vi "Find Center.vi"(5 "Position":i32, 7 "Tray Number":dbl format="%#_13g", 8 "Assembly Type":string, 9 "XYZTheta":dbl[](array[numeric]), 10 "component thickness":dbl, 11 "Gantry In":refnum<k24>) -> (0 "Pedestal Heights":dbl[][](array[numeric]), 1 "XYZTheta Centers":dbl[][](array[numeric]), 3 "Gantry Out":refnum<k24>)   [LabVIEW 2021, in "Assembly Tray.lvclass"]
uses:
  Assembly Tray.lvclass
  Find Tray.ctl
  Controller/Camera/Machine Vision.ctl
  C:/Program Files (x86)/Aerotech/A3200/LabVIEW/2010/Bin/Aerotech.A3200.dll
  Program Files (x86)/Aerotech/A3200/LabVIEW/2010/Bin/Aerotech.A3200.dll
  Controller/Camera/Image processing.ctl
  Controller/Camera/Camera settings.ctl
  <vilib>/Utility/file.llb/Read Delimited Spreadsheet (DBL).vi
  Controller/Camera/Camera.lvclass
  Controller/Motion/A3200/A3200.lvclass
  Controller/Motion/Motion.lvclass
  <vilib>/vision/NI_Vision_Development_Module.lvlib
panel:
  out "Global Report.Standard Variation":sgl
  in  "BP check":bool
  out "Program Done?":bool
  out "Manual Mode?":bool
  in  "Enter Manual Mode":bool
  out "error out":errorcluster
  out "Radius (Real-World)":dbl
  out "Match found?":bool
  out "Distance as expected?":bool
  in  "Auto Submit":bool
  out "Instructions":string="Use the joystick to match the pattern recognition until a red circle appears.\nUse Z controls to focus if needed."
  out "resulting string":string
  out "Current Z High Speed":dbl
  out "Current XY High Speed":dbl
  out "current Z low speed":dbl
  out "current XY speed":dbl
  in  "Z high":dbl=12.5
  in  "XY high":dbl=50.0
  in  "Z low":dbl=0.05
  in  "XY low":dbl=0.1
  out "Low Speed":bool
  out "X":bool
  out "Y":bool
  out "Z":bool
  out "High Speed":bool
  out "Move by":dbl[](array[numeric])
  in  "Autofiducial (Beta)":bool
  out "maximum is best focus":dbl
  in  "Focus":bool
  in  "Camera settings":T1={"Gamma"=1.6, "Gain"=0, "Sharpness"=0, "Contrast"=0.0, "Exposure"=0.0078125} {"Exposure" min=0.000244140625 max=0.5 scale=0.0002..0.5; "Contrast" min=0.0 max=1.0 scale=0.001..1.0; "Sharpness" min=0 max=2 step=1 scale=0.0..2.0; "Gain" min=0 max=100 step=1 scale=0.1..100.0; "Gamma" min=0.01 max=10.0 scale=0.01..10.0}
  in  "Image processing":T2={"Brightness"=128.0, "Contrast"=45.0, "Gamma"=1.0471123} {"Brightness" scale=0.0..400.0; "Contrast" scale=0.0..90.0; "Gamma" scale=0.005..5.0}
  in  "Override camera presets":bool
  out "Both fiducials recorded":bool
  in  "Machine Vision":T3
  out "Right Fiducial":dbl[](array[numeric]) format="%.6g"
  out "Left Fiducial":dbl[](array[numeric]) format="%.6g"
  out "Gantry":dbl[](array[numeric]) format="%.6g"
  out "Sum":dbl[](array[numeric]) format="%.6g"
  out "Camera":dbl[](array[numeric]) format="%.6g"
  in  "Carrier Tray":T4
  out "Image":T5(plugin-control)
  out "Center":dbl[](array[numeric]) format="%.6g"
  in  "Position Number":i16=1
  in  "Go to Center":bool
  in  "Calculate":bool
  in  "Record Top Right":bool
  in  "Record Top Left":bool
  in  "Go to Top Right Fiducial":bool
  in  "Go to Top Left Fiducial":bool
  in  "Joystick":bool
  in  "Stop":bool
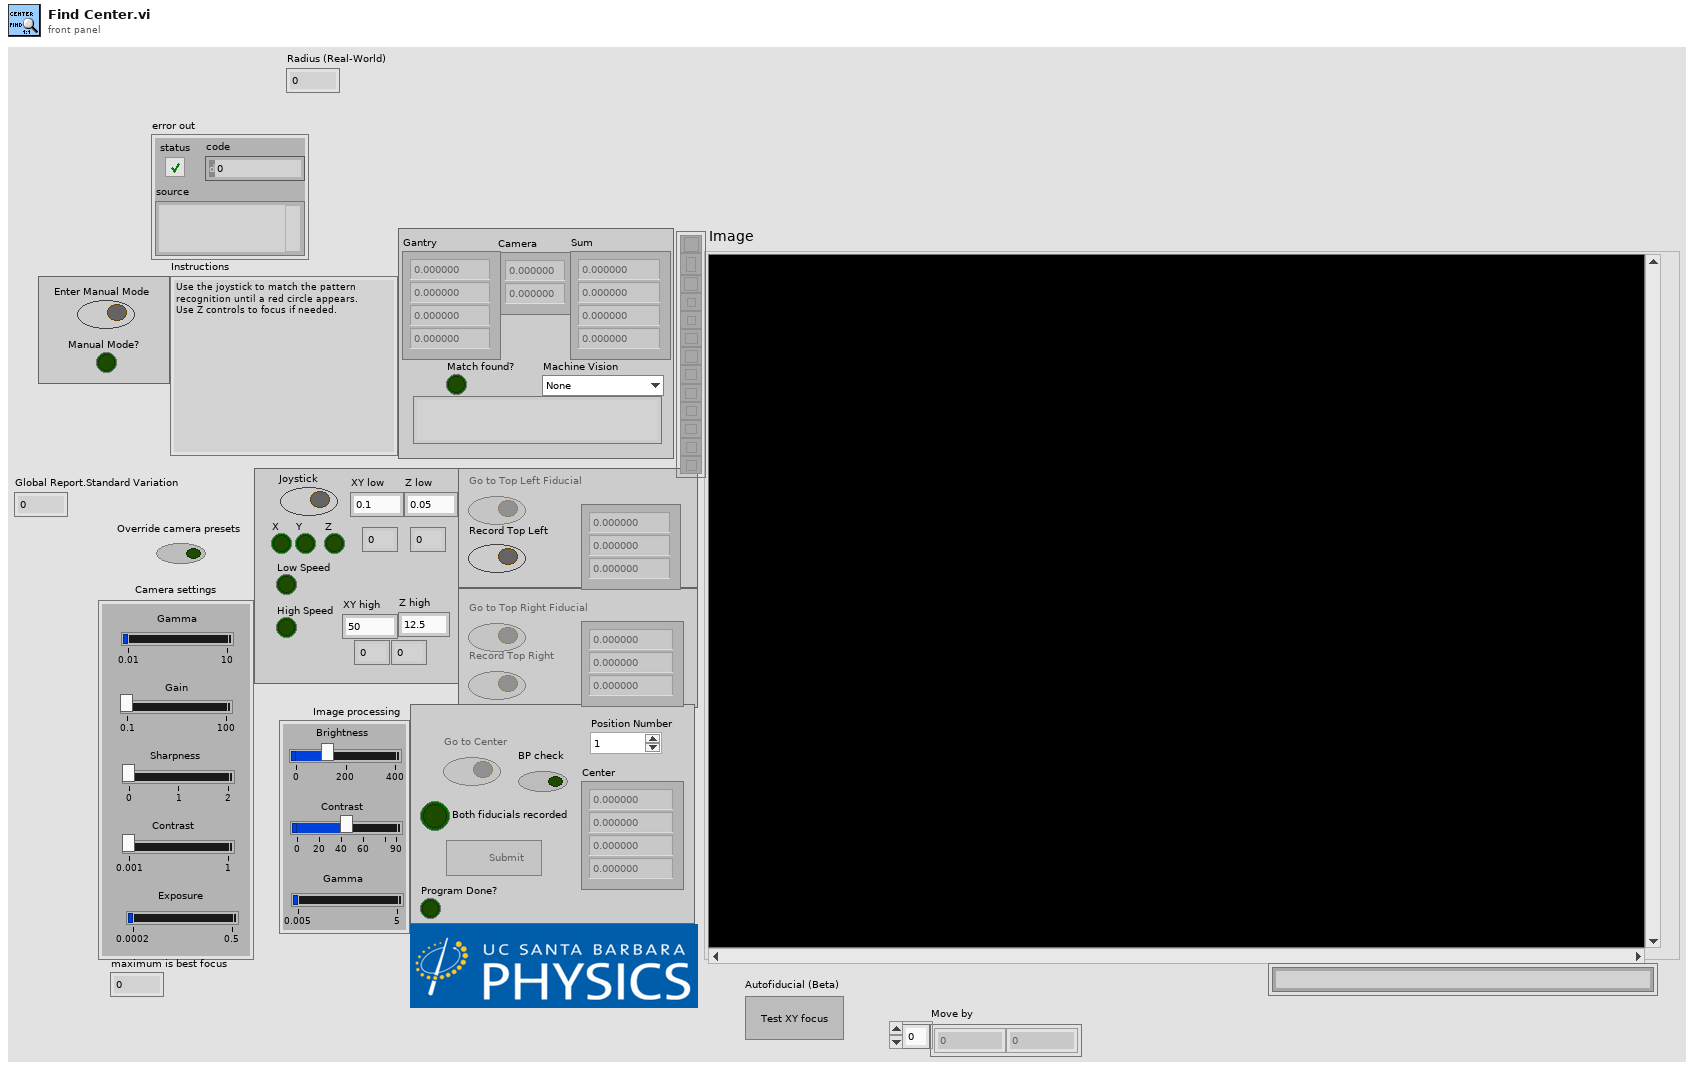
[diagram p1: front panel]
types:
  T1 = typedef "Camera.lvclass/Camera settings.ctl" = cluster{"Gamma":dbl, "Gain":i64, "Sharpness":i64, "Contrast":dbl, "Exposure":dbl}
  T2 = typedef "Camera.lvclass/Image processing.ctl" = cluster{"Brightness":sgl, "Contrast":sgl, "Gamma":sgl}
  T3 = typedef "Camera.lvclass/Machine Vision.ctl" = enum16{"None", "Assembly Tray Circle", "Assembly Tray Fiducial", "Partial Hexaboard", "sensor edge init", "HB edge init", "sensor edge pos1", "sensor edge pos2", "HB edge pos1", "HB edge pos2", "Sensor CH1-2", "HB CH1", "HB CH2", "V3 Sensor Circle", "Hexaboard Circle", "sensor CH1 check", "HB CH1 check ", "sensor ID"}
  T4 = typedef "Assembly Tray.lvclass/Find Tray.ctl" = cluster{"Gantry Fiducials":dbl[], "Relative Coordinates":dbl[][], "Camera Fiducials":dbl[][], "XYZTheta Centers":dbl[][], "Workspace Center":dbl[], "Syringe Relative Coordinates":dbl[], "Gantry Region":dbl, "Fiducials":path, "New Fiducials":dbl[][], "Past Fiducials":dbl[][], "XYZTheta":dbl[], "Pedestal Heights":dbl[][], "Assembly Type":string, "Tray Number":string, "Position":i32, "Protomodule?":bool, "avg value count":dbl[], "Previous Avgs":dbl[][], "Offset pins":dbl[][]}
  T5 = typedef "IMAQ Image.ctl" = refnum<image>
  T6 = cluster{"Average Strength":dbl, "Radius (Real-World)":dbl, "Match found?":bool, "initial angle":sgl, "Global Report":cluster{"Mean Value":sgl, "Standard Variation":sgl, "Minimal Value":sgl, "Maximal Value":sgl, "Area (calibrated)":sgl, "Area (pixels)":u32, "%":sgl, "Calibration Valid":bool}}
  T7 = enum8{"Enabled", "Disabled", "Disabled and Grayed Out"}
  T8 = typedef "File Paths.ctl" = cluster{"Glue Pattern Folder":path, "Carrier Tray Folder":path, "Pick Up Tool Fixture Folder":path, "Components Folder":path, "Bellows Tool Offset.txt":path, "Pick Up Tool Offset.txt":path, "Dispense Tip Offset.txt":path, "Log Files":path, "Gantry Assembly Map.txt":path, "Syringe and offset map.txt":path, "Controllers Folder":path, "Local dbase config":path}
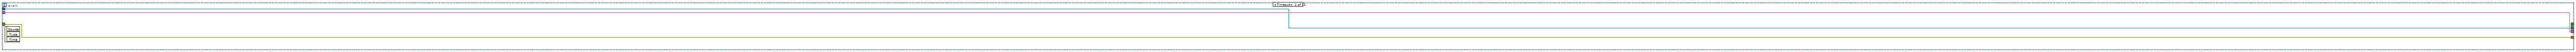
[diagram p3: hidden frame]
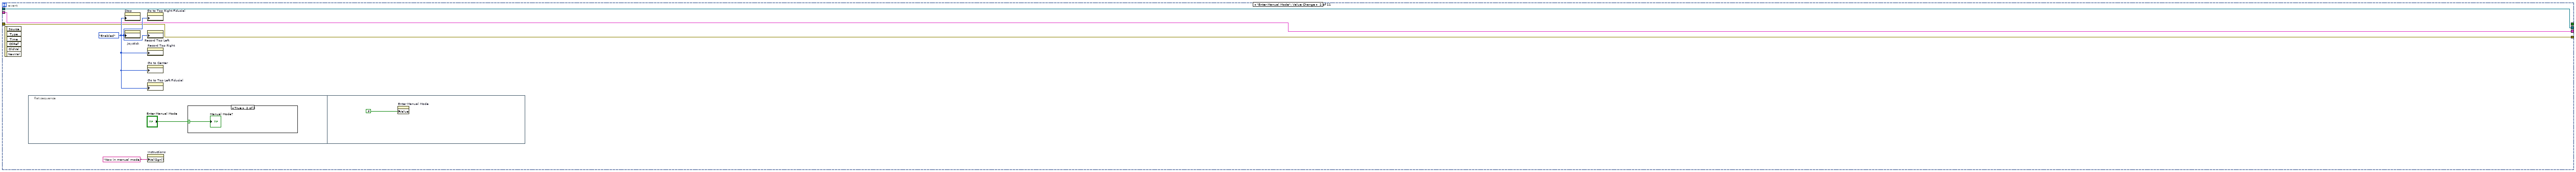
[diagram p4: hidden frame]
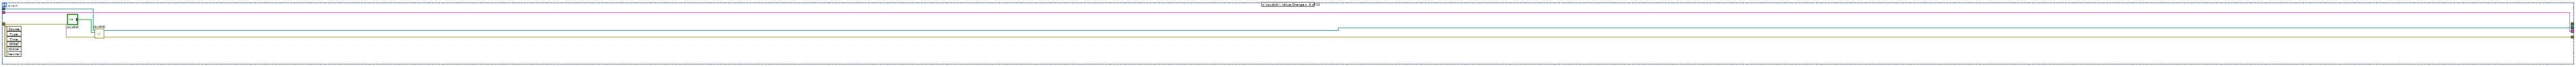
[diagram p6: hidden frame]
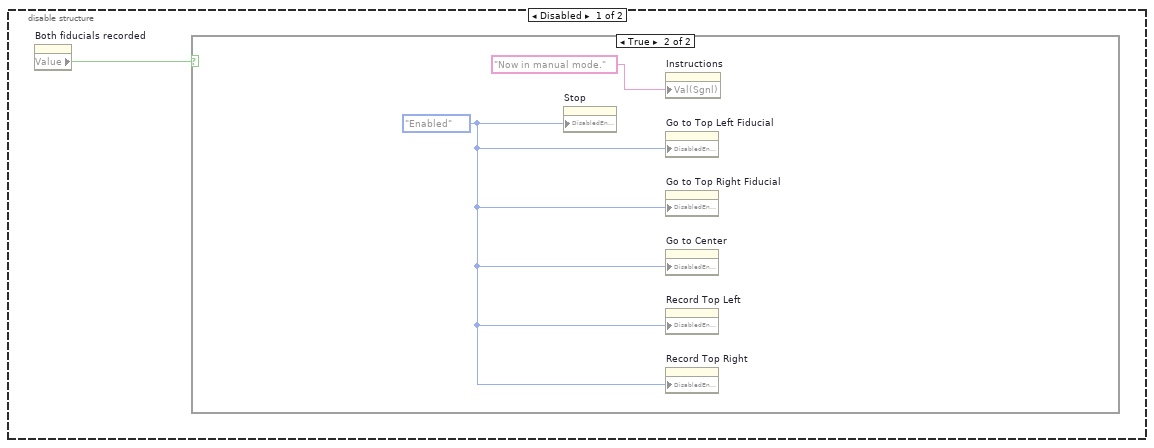
[diagram p7: hidden frame]
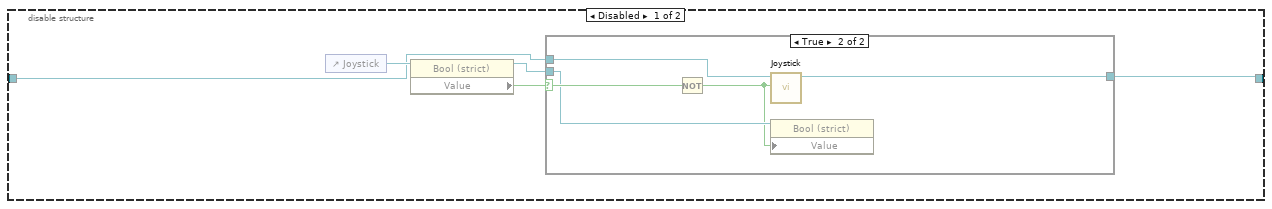
[diagram p9: hidden frame]
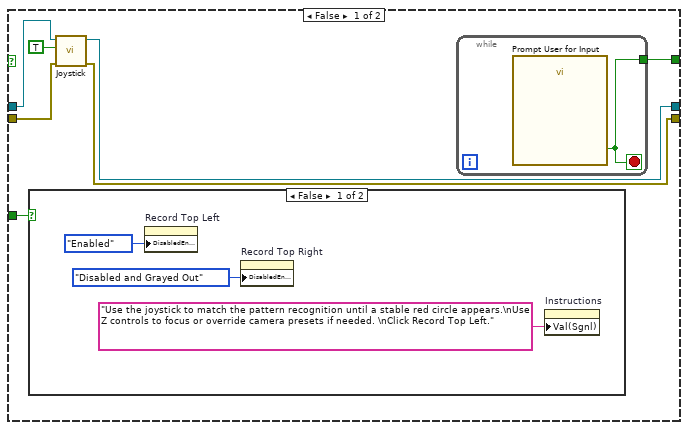
[diagram p12: hidden frame]
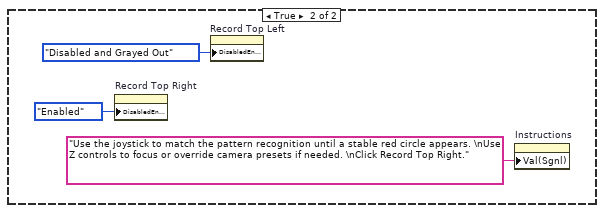
[diagram p13: hidden frame]
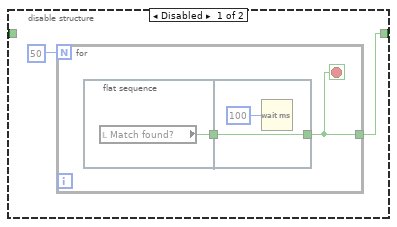
[diagram p19: hidden frame]
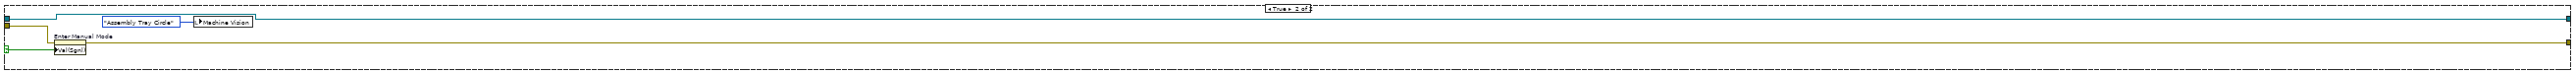
[diagram p20: hidden frame]
diagram:
  n1 = flat-sequence {
    tunnel: [w17] -> w9
    tunnel: ["Gantry In"] -> w8
    tunnel: [w16] -> w7
    tunnel: [w14] -> w4
    tunnel: [w29] -> w5
    tunnel: w9 -> [w29]
    tunnel: [w27] -> w2
    tunnel: w8 -> [w27]
    tunnel: w7 -> [w26]
    tunnel: [w26] -> w6
    tunnel: [w25] -> w1
    tunnel: w4 -> [w24]
    frame #0 {
      n2 = Decrement(x="Position") -> (x-1=w21:i32)
      n3 = call "Find Center Setup.vi"("XYZTheta"="XYZTheta", "Assembly Type"="Assembly Type", "Position"=w21, "Tray Number"="Tray Number", "Carrier Tray"="Carrier Tray") -> ("Assembly Tray Out"=w17:T4)  [unwired: 6 in]
      n4 = call "Get Camera Object.vi"() -> ("error out"=w14:errorcluster, "Camera out"=w16:refnum<class "Camera.lvclass">)  [unwired: 10 in]
    }
    frame #1 {
      n5 = control-ref of="This VI"() -> (w28:refnum<vi>)
      n6 = invoke class="VI" method="Default Vals.Reinit All"(reference=w28, error in=w24) -> (error out=w25:errorcluster)  [unwired: 1 in, 2 out]
    }
  }
  n7 = while {
    shift-right: [w36] -> _
    shift-left: w6 -> [w37]
    tunnel: w2 -> [w34]
    shift-right: [w33] -> _
    shift-left: _ -> [_]
    shift-right: [w31] -> _
    shift-left: w1 -> [w32]
    i -> [w35]
    stop <- w30 stop-if-true
    n8 = flat-sequence {
      tunnel: [w58] -> w36
      tunnel: w34 -> [w44]
      tunnel: [w43] -> w33
      tunnel: w32 -> [w42]
      tunnel: [w41] -> w31
      tunnel: w37 -> [w61]
      tunnel: w35 -> [w56]
      tunnel: [w39] -> w30
      frame #0 {
        n9 = in-place {
          in-place-border: w44 -> [w88]
          in-place-border: [w69] -> w47
          in-place-border: w42 -> [w64]
          in-place-border: [w62] -> w48
          # "Joystck Status"
          n10 = call "Get Joytick Status.vi"("error in (no error)"=w64, "Gantry In"=w88) -> ("error out"=w63:errorcluster, "JoystickLowSpeedActive"=w82:bool, "Joystick Status"=w84:bool[], "Gantry Out"=w70:refnum<k24>, "High Speeds"=w66:dbl[], "Low Speeds"=w65:dbl[])  [unwired: 4 in]
          n11 = Build Array("XY low", "XY low", "XY low", "Z low") -> (w68:dbl[])
          n12 = Build Array("XY high", "XY high", "XY high", "Z high") -> (w67:dbl[])
          n13 = call "Set Joystick Speed.vi"("error in (no error)"=w63, "High Speed Inputs"=w67, "Low Speed Inputs"=w68, "Gantry"=w70) -> ("error out"=w62:errorcluster, "Controller Out"=w69:refnum<k24>)  [unwired: 6 in]
          n14 = Or Array Elements(Boolean array=w84) -> (logical OR=w80:bool)
          n15 = Not(x=w82) -> (.not. x?=w81:bool)
          n16 = Index Array(array=w66) -> (element #1=→"Current XY High Speed":dbl, element #3=→"Current Z High Speed":dbl)  [unwired: 3 in, 1 out]
          n17 = Index Array(array=w65) -> (element #1=→"current XY speed":dbl, element #3=→"current Z low speed":dbl)  [unwired: 3 in, 1 out]
          n18 = Index Array(array=w84) -> (element #1=→"X":bool, element #2=→"Y":bool, element #3=→"Z":bool)  [unwired: 3 in]
          n19 = And(x=w80, y=w82) -> (x .and. y?=→"Low Speed":bool)
          n20 = And(x=w81, y=w80) -> (x .and. y?=→"High Speed":bool)
        }
        n21 = Equal To 0?(x=w56) -> (x = 0?=w55:bool)
        n22 = local read "Program Done?"() -> (w39:bool)
        n23 = call "Camera.vi"("Camera in"=w61, "Stop"=w39, "BCG Image Processing"="Image processing", "Machine Vision"="Machine Vision", "Camera settings"="Camera settings", "Loop 0"=w55, "Override presets"="Override camera presets") -> ("Camera out"=w58:refnum<class "Camera.lvclass">, "output cluster"=w54:T6, "Image"=→"Image":T5, "Camera"=w40:dbl[])  [unwired: 5 in, 4 out]
        "Camera" <- w40
        n24 = call "Get Current Position.vi"("error in (no error)"=w48, "Gantry In"=w47) -> ("error out"=w41:errorcluster, "XYZTheta Out"=w46:dbl[], "Gantry Out"=w43:refnum<k24>)  [unwired: 7 in]
        "Gantry" <- w46
        n25 = Unbundle By Name(w54) -> ("Average Strength"=→"maximum is best focus":dbl, "Radius (Real-World)"=→"Radius (Real-World)":dbl, "Match found?"=→"Match found?":bool, "Global Report.Standard Variation"=w38:sgl)
        "Global Report.Standard Variation" <- w38
        n26 = shared-variable ".\\Assembly Tray.lvclass\\BP Standard Variation"(w38) -> ()  [unwired: 1 in, 1 out]
        n27 = Add(x=w46, y=w40) -> (x+y=→"Sum":dbl[])
      }
    }
  }
  n28 = while {
    shift-right: [w98] -> w13
    shift-left: w5 -> [w99]
    shift-right: [w95] -> w11
    shift-left: w2 -> [w96]
    tunnel: w5 -> [w91]
    shift-right: [w89] -> w3
    shift-left: w1 -> [w90]
    i -> [w94]
    stop <- w97 stop-if-true
    n29 = event shown="[3] \"Go to Top Left Fiducial\", \"Go to Top Right Fiducial\": Value Change" {
      selector: _ -> [_ _ _ _ _ _ _ _ _ _ _]
      dyn-events: _ -> [_ _ _ _ _ _ _ _ _ _ _]
      timeout: _ -> [_ _ _ _ _ _ _ _ _ _ _]
      tunnel: [w111 w114 w125 w143 w366 w425 w563 w711 w789 w809 w882] -> w98
      tunnel: w99 -> [w111 w114 w125 w143 w362 w425 w564 w711 w790 w809 w882]
      tunnel: [_ _ _ _ _ _ _ _ _ w810 _] -> w97
      tunnel: w96 -> [w110 w115 w124 w142 w361 w424 w569 w721 w787 w813 w884]
      tunnel: [w110 w115 w122 w141 w360 w423 w569 w714 w784 w812 w885] -> w95
      tunnel: [w109 w113 w120 w132 w355 w419 w557 w715 w781 w817 w880] -> w89
      tunnel: w90 -> [w109 w113 w121 w133 w357 w418 w560 w720 w781 w814 w881]
      event Timeout {
        n30 = event-data() -> ()  [unwired: 1 in, 3 out]
      }
      event "Enter Manual Mode": Value Change {
        w116 = T7."Enabled" ("Disabled")
        n31 = event-data() -> ()  [unwired: 1 in, 6 out]
        n32 = flat-sequence {
          frame #0 {
            n33 = case shown="True" "Enter Manual Mode" {
              selector: "Enter Manual Mode" -> [_ w118]
              frame False {
              }
              frame True {
                "Manual Mode?" <- w118
              }
            }
          }
          frame #1 {
            n34 = property on="Enter Manual Mode" class="Bool (strict)"("Value"=FALSE ("Enter Manual Mode")) -> ()  [unwired: 2 in, 2 out]
          }
        }
        n35 = property on="Stop" class="Bool"("DisabledEnum"=w116) -> ()  [unwired: 2 in, 2 out]
        n36 = property on="Joystick" class="Bool (strict)"("DisabledEnum"=w116) -> ()  [unwired: 2 in, 2 out]
        n37 = property on="Go to Top Right Fiducial" class="Bool (strict)"("DisabledEnum"=w116) -> ()  [unwired: 2 in, 2 out]
        n38 = property on="Record Top Left" class="Bool (strict)"("DisabledEnum"=w116) -> ()  [unwired: 2 in, 2 out]
        n39 = property on="Record Top Right" class="Bool (strict)"("DisabledEnum"=w116) -> ()  [unwired: 2 in, 2 out]
        n40 = property on="Go to Center" class="Bool"("DisabledEnum"=w116) -> ()  [unwired: 2 in, 2 out]
        n41 = property on="Go to Top Left Fiducial" class="Bool (strict)"("DisabledEnum"=w116) -> ()  [unwired: 2 in, 2 out]
        n42 = property on="Instructions" class="Str"("Val(Sgnl)"="Now in manual mode." ("Value (Signaling)")) -> ()  [unwired: 2 in, 2 out]
      }
      event "Joystick": Value Change {
        n43 = event-data() -> ()  [unwired: 1 in, 6 out]
        n44 = call "Joystick.vi"("error in (no error)"=w121, "Joystick"="Joystick", "Gantry In"=w124) -> ("error out"=w120:errorcluster, "Gantry Out"=w122:refnum<k24>)  [unwired: 7 in]
      }
      event "Go to Top Left Fiducial", "Go to Top Right Fiducial": Value Change {
        n45 = event-data() -> ()  [unwired: 1 in, 6 out]
        n46 = disable-structure shown="Enabled" {
          frame Disabled {
            n47 = property on="Both fiducials recorded" class="Bool (strict)"() -> ("Value"=w144:bool)  [unwired: 2 in, 2 out]
            n48 = case shown="True" w144 {
              frame False {
              }
              frame True {
                w145 = T7."Enabled" ("Disabled")
                n49 = property on="Stop" class="Bool"("DisabledEnum"=w145) -> ()  [unwired: 2 in, 2 out]
                n50 = property on="Instructions" class="Str"("Val(Sgnl)"="Now in manual mode." ("Value (Signaling)")) -> ()  [unwired: 2 in, 2 out]
                n51 = property on="Go to Top Left Fiducial" class="Bool (strict)"("DisabledEnum"=w145) -> ()  [unwired: 2 in, 2 out]
                n52 = property on="Go to Top Right Fiducial" class="Bool (strict)"("DisabledEnum"=w145) -> ()  [unwired: 2 in, 2 out]
                n53 = property on="Go to Center" class="Bool"("DisabledEnum"=w145) -> ()  [unwired: 2 in, 2 out]
                n54 = property on="Record Top Left" class="Bool (strict)"("DisabledEnum"=w145) -> ()  [unwired: 2 in, 2 out]
                n55 = property on="Record Top Right" class="Bool (strict)"("DisabledEnum"=w145) -> ()  [unwired: 2 in, 2 out]
              }
            }
          }
          frame Enabled {
          }
        }
        n56 = disable-structure shown="Enabled" {
          disable-tunnel: w142 -> [w149 w158]
          disable-tunnel: [w147 w158] -> w140
          frame Disabled {
            n57 = control-ref of="Joystick"() -> (w151:refnum<vi>)
            n58 = property class="Bool (strict)"(reference=w151) -> (reference out=w148:refnum<vi>, "Value"=w150:bool)  [unwired: 1 in, 1 out]
            n59 = case shown="True" w150 {
              selector: w150 -> [_ w157]
              tunnel: w149 -> [w152 w155]
              tunnel: [w152 w154] -> w147
              tunnel: w148 -> [_ w156]
              frame False {
              }
              frame True {
                n60 = Not(x=w157) -> (.not. x?=w153:bool)
                n61 = call "Joystick.vi"("Joystick"=w153, "Gantry In"=w155) -> ("Gantry Out"=w154:refnum<k24>)  [unwired: 8 in, 1 out]
                n62 = property class="Bool (strict)"(reference=w156, "Value"=w153) -> ()  [unwired: 1 in, 2 out]
              }
            }
          }
          frame Enabled {
          }
        }
        n63 = Unbundle By Name "Unbundle By Name"(w143) -> ("Gantry Fiducials"=w135:dbl[])
        n64 = flat-sequence {
          tunnel: w135 -> [w160]
          tunnel: w140 -> [w161]
          tunnel: [w161] -> w131
          tunnel: [w160] -> w129
          tunnel: ["Go to Top Right Fiducial"] -> w127
          tunnel: ["Go to Top Right Fiducial"] -> w134
          tunnel: w131 -> [w165]
          tunnel: [w165] -> w130
          tunnel: w129 -> [w164]
          tunnel: [w164] -> w128
          tunnel: w127 -> [w163]
          tunnel: [w163] -> w126
          tunnel: [w183] -> w139
          tunnel: [w179] -> w136
          tunnel: w130 -> [w177]
          tunnel: w128 -> [w174]
          tunnel: w126 -> [w171]
          tunnel: w133 -> [w167]
          tunnel: w139 -> [w185]
          tunnel: [w185] -> w138
          tunnel: [w184] -> w137
          tunnel: w136 -> [w184]
          tunnel: [w188] -> w141
          tunnel: [w187] -> w132
          tunnel: w137 -> [w190]
          tunnel: w134 -> [w191]
          tunnel: w138 -> [w192]
          frame #0 {
          }
          frame #1 {
            w162 = FALSE ("Go to Top Right Fiducial")
            n65 = property on="Go to Top Left Fiducial" class="Bool (strict)"("Value"=w162) -> ()  [unwired: 2 in, 2 out]
            n66 = property on="Go to Top Right Fiducial" class="Bool (strict)"("Value"=w162) -> ()  [unwired: 2 in, 2 out]
          }
          frame #2 {
            w180 = T7."Disabled and Grayed Out" ("Disabled")
            n67 = Select(t=3, s=w171, f=0) -> (s? t:f=w169:i32)
            n68 = call "Joystick.vi"("error in (no error)"=w167, "Joystick"=FALSE, "Gantry In"=w177) -> ("error out"=w175:errorcluster, "Gantry Out"=w178:refnum<k24>)  [unwired: 7 in]
            n69 = Array Subset "Array Subset"(array=w174, index=w169, length=3) -> (w173:dbl[])
            n70 = property on="Instructions" class="Str"("Val(Sgnl)"="Wait for movement to stop." ("Value (Signaling)")) -> ()  [unwired: 2 in, 2 out]
            n71 = property on="Go to Center" class="Bool"("DisabledEnum"=w180) -> ()  [unwired: 2 in, 2 out]
            n72 = property on="Stop" class="Bool"("DisabledEnum"=w180) -> ()  [unwired: 2 in, 2 out]
            n73 = property on="Record Top Right" class="Bool (strict)"("DisabledEnum"=w180) -> ()  [unwired: 2 in, 2 out]
            n74 = property on="Go to Top Right Fiducial" class="Bool (strict)"("DisabledEnum"=w180) -> ()  [unwired: 2 in, 2 out]
            n75 = property on="Go to Top Left Fiducial" class="Bool (strict)"("DisabledEnum"=w180) -> ()  [unwired: 2 in, 2 out]
            n76 = property on="Record Top Left" class="Bool (strict)"("DisabledEnum"=w180) -> ()  [unwired: 2 in, 2 out]
            n77 = local write "Machine Vision"(Machine_Vision."Assembly Tray Fiducial" ("Machine Vision")) -> ()
            n78 = call "ClearXYZTheta Go.vi"("error in (no error)"=w175, "Speed"=300.0, "XYZTheta In"=w173, "Gantry In"=w178) -> ("error out"=w179:errorcluster, "Gantry Out"=w183:refnum<k24>)  [unwired: 5 in, 1 out]
          }
          frame #3 {
            n79 = disable-structure shown="Enabled" {
              frame Enabled {
                n80 = Wait (ms)(milliseconds to wait=u32 500) -> ()  [unwired: 1 out]
              }
              frame Disabled {
              }
            }
          }
          frame #4 {
            n81 = local read "Manual Mode?"() -> (w189:bool)
            n82 = case shown="False" w189 {
              selector: w189 -> [_ w352]
              tunnel: w192 -> [w214 w353]
              tunnel: [w194 w353] -> w188
              tunnel: w191 -> [w195 _]
              tunnel: w190 -> [w213 w351]
              tunnel: [w193 w350] -> w187
              frame False {
                n83 = flat-sequence {
                  tunnel: w214 -> [w239]
                  tunnel: w213 -> [w237]
                  tunnel: [w238] -> w212
                  tunnel: [w236] -> w211
                  tunnel: [w235] -> w210
                  tunnel: [w234] -> w209
                  tunnel: w212 -> [w299]
                  tunnel: w211 -> [w298]
                  tunnel: w210 -> [w297]
                  tunnel: w209 -> [w296]
                  tunnel: [w299] -> w208
                  tunnel: [w298] -> w206
                  tunnel: [w297] -> w204
                  tunnel: [w296] -> w202
                  tunnel: w208 -> [w303]
                  tunnel: [w303] -> w207
                  tunnel: w206 -> [w302]
                  tunnel: [w302] -> w205
                  tunnel: w204 -> [w301]
                  tunnel: [w301] -> w203
                  tunnel: w202 -> [w300]
                  tunnel: [w300] -> w201
                  tunnel: w207 -> [w311]
                  tunnel: w205 -> [w310]
                  tunnel: w203 -> [w306]
                  tunnel: w201 -> [w309]
                  tunnel: [w308] -> w199
                  tunnel: [w307] -> w200
                  tunnel: [w305] -> w196
                  frame #0 {
                    n84 = for {
                      N: 50 -> [_]
                      tunnel: [w242] -> w240
                      tunnel: [w241] -> w232
                      stop <- w242 stop-if-true
                      n85 = flat-sequence {
                        tunnel: [w245] -> w243
                        tunnel: [w244] -> w241
                        tunnel: [w247] -> w242
                        tunnel: w243 -> [w247]
                        frame #0 {
                          n86 = local read "Match found?"() -> (w245:bool)
                          n87 = local read "Camera"() -> (w244:dbl[])
                        }
                        frame #1 {
                          n88 = Wait (ms)(milliseconds to wait=u32 100) -> ()  [unwired: 1 out]
                        }
                      }
                    }
                    n89 = case shown="False" w240 {
                      selector: w240 -> [_ w292]
                      tunnel: w239 -> [w251 w294]
                      tunnel: [w253 w294] -> w238
                      tunnel: w237 -> [w250 w293]
                      tunnel: [w252 w293] -> w236
                      tunnel: [w249 w292] -> w235
                      tunnel: [w248 w291] -> w234
                      tunnel: w232 -> [_ w291]
                      frame False {
                        n90 = flat-sequence {
                          tunnel: [w265] -> w253
                          tunnel: [w264] -> w252
                          tunnel: w251 -> [w263]
                          tunnel: w250 -> [w262]
                          tunnel: [w257] -> w249
                          tunnel: [w254] -> w248
                          frame #0 {
                            n91 = call "Base File Path.vi"() -> ("Paths Out"=w259:T8)  [unwired: 11 in]
                            n92 = Unbundle By Name(w259) -> ("Controllers Folder"=w260:path)
                            n93 = String To Path(string="Scan.txt") -> (path=w261:path)
                            n94 = Build Path(base path=w260, name or relative path=w261) -> (appended path=w256:path)
                            n95 = call-poly <vilib>:"Read Delimited Spreadsheet.vi"("file path (dialog if empty)"=w256) -> ("all rows"=w255:dbl[][])  [unwired: 9 in, 5 out]
                            n96 = for {
                              shift-right: [w275] -> w265
                              shift-left: w263 -> [w276]
                              tunnel: w255 -> [w274] mode=indexing
                              shift-right: [w272] -> w264
                              shift-left: w262 -> [w273]
                              tunnel: [w267] -> w257
                              tunnel: [w266] -> w254
                              stop <- w267 stop-if-true
                              n97 = flat-sequence {
                                tunnel: w276 -> [w283]
                                tunnel: w274 -> [w281]
                                tunnel: w273 -> [w279]
                                tunnel: [w282] -> w271
                                tunnel: [w278] -> w270
                                tunnel: w271 -> [w284]
                                tunnel: w270 -> [w285]
                                tunnel: [w284] -> w269
                                tunnel: [w285] -> w268
                                tunnel: [w289] -> w272
                                tunnel: [w290] -> w275
                                tunnel: w269 -> [w290]
                                tunnel: w268 -> [w289]
                                tunnel: [w288] -> w267
                                tunnel: [w287] -> w266
                                frame #0 {
                                n98 = call "XY Go.vi"("Increment?"=TRUE, "error in (no error)"=w279, "Speed"=0.1, "XY In"=w281, "Gantry In"=w283) -> ("error out"=w278:errorcluster, "Gantry Out"=w282:refnum<k24>)  [unwired: 4 in, 1 out]
                                }
                                frame #1 {
                                n99 = disable-structure shown="Enabled" {
                                disable-tunnel: w284 -> [_ _]
                                frame Enabled {
                                n100 = Wait (ms)(milliseconds to wait=u32 500) -> ()  [unwired: 1 out]
                                }
                                frame Disabled {
                                }
                                }
                                }
                                frame #2 {
                                n101 = local read "Match found?"() -> (w288:bool)
                                n102 = local read "Camera"() -> (w287:dbl[])
                                }
                              }
                            }
                          }
                        }
                      }
                      frame True {
                      }
                    }
                  }
                  frame #1 {
                    n103 = local write "Machine Vision"(Machine_Vision."Assembly Tray Circle" ("Machine Vision")) -> ()
                  }
                  frame #2 {
                    n104 = disable-structure shown="Enabled" {
                      frame Enabled {
                        n105 = Wait (ms)(milliseconds to wait=u32 500) -> ()  [unwired: 1 out]
                      }
                      frame Disabled {
                      }
                    }
                  }
                  frame #3 {
                    n106 = case shown="True" w306 {
                      selector: w306 -> [w312 w315]
                      tunnel: w311 -> [w314 w325]
                      tunnel: [w314 w324] -> w308
                      tunnel: w310 -> [w313 w323]
                      tunnel: [w313 w322] -> w307
                      tunnel: w309 -> [_ w321]
                      tunnel: [w312 w316] -> w305
                      frame False {
                      }
                      frame True {
                        n107 = flat-sequence {
                          tunnel: w325 -> [w333]
                          tunnel: w323 -> [w331]
                          tunnel: w321 -> [w326]
                          tunnel: [w332] -> w320
                          tunnel: [w330] -> w319
                          tunnel: w320 -> [w335]
                          tunnel: w319 -> [w334]
                          tunnel: [w335] -> w318
                          tunnel: [w334] -> w317
                          tunnel: [w339] -> w322
                          tunnel: [w340] -> w324
                          tunnel: w318 -> [w340]
                          tunnel: w317 -> [w339]
                          tunnel: [w338] -> w316
                          tunnel: w315 -> [w337]
                          frame #0 {
                            n108 = call "XY Go.vi"("Increment?"=TRUE, "error in (no error)"=w331, "Speed"=5.0, "XY In"=w326, "Gantry In"=w333) -> ("error out"=w330:errorcluster, "Gantry Out"=w332:refnum<k24>)  [unwired: 4 in, 1 out]
                            n109 = property on="Instructions" class="Str"("Val(Sgnl)"="Fiducial found." ("Value (Signaling)")) -> ()  [unwired: 2 in, 2 out]
                          }
                          frame #1 {
                            n110 = disable-structure shown="Enabled" {
                              frame Enabled {
                                n111 = Wait (ms)(milliseconds to wait=u32 500) -> ()  [unwired: 1 out]
                              }
                              frame Disabled {
                              }
                            }
                          }
                          frame #2 {
                            n112 = disable-structure shown="Enabled" {
                              disable-tunnel: [w342 w348] -> w338
                              disable-tunnel: w337 -> [_ w348]
                              frame Disabled {
                                n113 = for {
                                N: 50 -> [_]
                                tunnel: [w343] -> w342
                                stop <- w343 stop-if-true
                                n114 = flat-sequence {
                                tunnel: [w345] -> w344
                                tunnel: [w347] -> w343
                                tunnel: w344 -> [w347]
                                frame #0 {
                                n115 = local read "Match found?"() -> (w345:bool)
                                }
                                frame #1 {
                                n116 = Wait (ms)(milliseconds to wait=u32 100) -> ()  [unwired: 1 out]
                                }
                                }
                                }
                              }
                              frame Enabled {
                              }
                            }
                          }
                        }
                      }
                    }
                  }
                }
                n117 = case shown="True" w196 {
                  selector: w196 -> [_ w231]
                  tunnel: [w216 w231] -> w198
                  tunnel: w199 -> [w220 w230]
                  tunnel: [w219 w230] -> w194
                  tunnel: w200 -> [w218 w229]
                  tunnel: [w217 w229] -> w197
                  tunnel: w195 -> [w215 _]
                  frame False {
                    n118 = case shown="False" w215 {
                      frame False {
                        n119 = property on="Record Top Left" class="Bool (strict)"("DisabledEnum"=T7."Enabled" ("Disabled")) -> ()  [unwired: 2 in, 2 out]
                        n120 = property on="Record Top Right" class="Bool (strict)"("DisabledEnum"=T7."Disabled and Grayed Out" ("Disabled")) -> ()  [unwired: 2 in, 2 out]
                        n121 = property on="Instructions" class="Str"("Val(Sgnl)"="Use the joystick to match the pattern recognition until a stable red circle appears.\nUse Z controls to focus or override camera presets if needed. \nClick Record Top Left.") -> ()  [unwired: 2 in, 2 out]
                      }
                      frame True {
                        n122 = property on="Record Top Right" class="Bool (strict)"("DisabledEnum"=T7."Enabled" ("Disabled")) -> ()  [unwired: 2 in, 2 out]
                        n123 = property on="Record Top Left" class="Bool (strict)"("DisabledEnum"=T7."Disabled and Grayed Out" ("Disabled")) -> ()  [unwired: 2 in, 2 out]
                        n124 = property on="Instructions" class="Str"("Val(Sgnl)"="Use the joystick to match the pattern recognition until a stable red circle appears. \nUse Z controls to focus or override camera presets if needed. \nClick Record Top Right.") -> ()  [unwired: 2 in, 2 out]
                      }
                    }
                    n125 = call "Joystick.vi"("error in (no error)"=w218, "Joystick"=TRUE, "Gantry In"=w220) -> ("error out"=w217:errorcluster, "Gantry Out"=w219:refnum<k24>)  [unwired: 7 in]
                    n126 = while {
                      tunnel: [w222] -> w216
                      stop <- w222 stop-if-true
                      n127 = call "Prompt User for Input"() -> ("Target line up?"=w222:bool)  [unwired: 17 in, 2 out]
                    }
                  }
                  frame True {
                  }
                }
                n128 = property on="Focus" class="Bool (strict)"(error in=w197, "Val(Sgnl)"=w198) -> (error out=w193:errorcluster)  [unwired: 1 in, 1 out]
              }
              frame True {
                n129 = property on="Enter Manual Mode" class="Bool (strict)"(error in=w351, "Val(Sgnl)"=w352) -> (error out=w350:errorcluster)  [unwired: 1 in, 1 out]
                n130 = local write "Machine Vision"(Machine_Vision."Assembly Tray Circle" ("Machine Vision")) -> ()
              }
            }
          }
        }
      }
      event "Record Top Left", "Record Top Right": Value Change {
        n131 = event-data() -> ()  [unwired: 1 in, 6 out]
        n132 = flat-sequence {
          tunnel: ["Record Top Right"] -> w354
          frame #0 {
          }
          frame #1 {
            w368 = FALSE ("Record Top Left")
            n133 = property on="Record Top Left" class="Bool (strict)"("Value"=w368) -> ()  [unwired: 2 in, 2 out]
            n134 = property on="Record Top Right" class="Bool (strict)"("Value"=w368) -> ()  [unwired: 2 in, 2 out]
          }
        }
        n135 = Boolean To (0,1)(Boolean=w354) -> (0, 1=w363:i16)
        n136 = in-place {
          in-place-border: [w387] -> w364
          in-place-border: w363 -> [w380]
          in-place-border: w361 -> [w382]
          in-place-border: [w381] -> w360
          in-place-border: w357 -> [w375]
          in-place-border: [w373] -> w356
          n137 = in-place-cluster #1(w362) -> ("Gantry Fiducials"=w384:dbl[], "Camera Fiducials"=w391:dbl[][])
          n138 = call "Get Current Position.vi"("error in (no error)"=w375, "Gantry In"=w382) -> ("error out"=w374:errorcluster, "XYZTheta Out"=w385:dbl[], "Gantry Out"=w381:refnum<k24>)  [unwired: 7 in]
          n139 = Multiply(x=w380, y=i16 3) -> (x*y=w378:i16)
          n140 = Reshape Array(w385, 3 ("dimension size")) -> (w377:dbl[])
          n141 = Replace Array Subset(array=w384, new element=w377, index=w378) -> (w383:dbl[])
          n142 = in-place {
            n143 = in-place-array #2(w377, 0, 1) -> (w399:dbl, w397:dbl)
            n144 = local read "Camera"() -> (w400:dbl[])
            n145 = Index Array(array=w400) -> (element #1=w398:dbl, element #2=w396:dbl)  [unwired: 2 in]
            n146 = Add(x=w399, y=w398) -> (x+y=w394:dbl)
            n147 = Add(x=w397, y=w396) -> (x+y=w395:dbl)
            n148 = in-place-array #2(w394, w395) -> (w376:dbl[])  [unwired: 2 out]
          }
          n149 = Reshape Array(w391, 2 ("length"), 3 ("dimension size")) -> (w390:dbl[][])
          n150 = case shown="0, Default" w380 {
            tunnel: w376 -> [w404 w416]
            tunnel: w374 -> [w403 w415]
            tunnel: [w402 w415] -> w373
            frame 0, Default {
              n151 = local read "Manual Mode?"() -> (w401:bool)
              n152 = case shown="True" w401 {
                selector: w401 -> [_ w414]
                tunnel: w403 -> [w406 w413]
                tunnel: [w405 w412] -> w402
                frame False {
                  n153 = property on="Both fiducials recorded" class="Bool (strict)"() -> ("Value"=w407:bool)  [unwired: 2 in, 2 out]
                  n154 = case shown="False" w407 {
                    tunnel: w406 -> [w409 w411]
                    tunnel: [w408 w411] -> w405
                    frame False {
                      n155 = property on="Go to Top Right Fiducial" class="Bool (strict)"(error in=w409, "Val(Sgnl)"=TRUE ("Value (Signaling)")) -> (error out=w408:errorcluster)  [unwired: 1 in, 1 out]
                    }
                    frame True {
                    }
                  }
                }
                frame True {
                  n156 = property on="Enter Manual Mode" class="Bool (strict)"(error in=w413, "Val(Sgnl)"=w414) -> (error out=w412:errorcluster)  [unwired: 1 in, 1 out]
                }
              }
              "Left Fiducial" <- w404
            }
            frame 1 {
              "Right Fiducial" <- w416
            }
          }
          n157 = Replace Array Subset(array=w390, new element=w376, index (row)=w380) -> (w387:dbl[][])  [unwired: 1 in]
          n158 = in-place-cluster #1("Gantry Fiducials"=w383, "Camera Fiducials"=w387) -> (w366:T4)
        }
        n159 = Multiply Array Elements(1:w364) -> (0:w365:dbl)
        n160 = Equal To 0?(x=w365) -> (x = 0?=w359:bool)
        n161 = Not(x=w359) -> (.not. x?=→"Both fiducials recorded":bool)
        n162 = case shown="False" w359 {
          selector: w359 -> [w371 _]
          tunnel: w356 -> [w370 w372]
          tunnel: [w369 w372] -> w355
          frame False {
            n163 = property on="Calculate" class="Bool (strict)"(error in=w370, "Val(Sgnl)"=w371) -> (error out=w369:errorcluster)  [unwired: 1 in, 1 out]
          }
          frame True {
          }
        }
      }
      event "Focus": Value Change {
        n164 = event-data() -> ()  [unwired: 1 in, 6 out]
        n165 = flat-sequence {
          tunnel: w418 -> [w428]
          tunnel: [w426] -> w417
          tunnel: w424 -> [w433]
          tunnel: [w432] -> w422
          tunnel: [w431] -> w421
          tunnel: [w430] -> w420
          tunnel: w417 -> [w429]
          tunnel: [w522] -> w423
          tunnel: w422 -> [w523]
          tunnel: w421 -> [w525]
          tunnel: w420 -> [w524]
          tunnel: [w521] -> w419
          frame #0 {
            n166 = property on="Focus" class="Bool (strict)"(error in=w428, "Value"=FALSE ("Focus")) -> (error out=w426:errorcluster)  [unwired: 1 in, 1 out]
          }
          frame #1 {
            n167 = local read "Match found?"() -> (w434:bool)
            n168 = case shown="False" w434 {
              tunnel: w433 -> [w462 w518]
              tunnel: [w450 w518] -> w432
              tunnel: [w451 w517] -> w431
              tunnel: w429 -> [w436 w517]
              tunnel: [w439 FALSE ("empty?")] -> w430
              frame False {
                n169 = property on="Instructions" class="Str"(error in=w436, "Val(Sgnl)"="Now finding best focus." ("Value (Signaling)")) -> (error out=w435:errorcluster)  [unwired: 1 in, 1 out]
                n170 = call "Joystick.vi"("error in (no error)"=w435, "Joystick"=FALSE, "Gantry In"=w462) -> ("error out"=w443:errorcluster, "Gantry Out"=w447:refnum<k24>)  [unwired: 7 in]
                n171 = call "Get Current Position.vi"("error in (no error)"=w443, "Gantry In"=w447) -> ("error out"=w445:errorcluster, "XYZTheta Out"=w444:dbl[], "Gantry Out"=w446:refnum<k24>)  [unwired: 7 in]
                n172 = call "Z Go.vi"("Increment"=TRUE, "Return Immediately"=FALSE ("Increment"), "error in (no error)"=w445, "Speed In"=1.0 ("Speed"), "Position In"=-0.1, "Gantry In"=w446) -> ("error out"=w458:errorcluster, "Gantry Out"=w461:refnum<k24>)  [unwired: 2 in, 2 out]
                n173 = for {
                  N: 20 -> [_]
                  shift-right: [w481] -> w452
                  shift-left: w461 -> [w483]
                  shift-right: [w480] -> w466
                  shift-left: dbl[][] [] -> [w473]
                  shift-right: [w477] -> w454
                  shift-left: w458 -> [w479]
                  n174 = flat-sequence {
                    tunnel: w483 -> [w486]
                    tunnel: [w486] -> w482
                    tunnel: w479 -> [w485]
                    tunnel: [w485] -> w478
                    tunnel: w482 -> [w493]
                    tunnel: w478 -> [w490]
                    tunnel: [w492] -> w476
                    tunnel: [w491] -> w475
                    tunnel: [w489] -> w474
                    tunnel: w473 -> [w487]
                    tunnel: [w509] -> w477
                    tunnel: [w515] -> w480
                    tunnel: [w510] -> w481
                    tunnel: w476 -> [w511]
                    tunnel: w475 -> [w515]
                    tunnel: w474 -> [w508]
                    frame #0 {
                      n175 = Wait (ms)(milliseconds to wait=u32 500) -> ()  [unwired: 1 out]
                    }
                    frame #1 {
                      n176 = local read "Match found?"() -> (w488:bool)
                      n177 = case shown="True" w488 {
                        tunnel: w493 -> [w495 w506]
                        tunnel: [w495 w505] -> w492
                        tunnel: [w494 w497] -> w491
                        tunnel: w490 -> [w496 w501]
                        tunnel: [w496 w500] -> w489
                        tunnel: w487 -> [w494 _]
                        frame False {
                        }
                        frame True {
                          n178 = call "Get Current Position.vi"("error in (no error)"=w501, "Gantry In"=w506) -> ("error out"=w500:errorcluster, "XYZTheta Out"=w504:dbl[], "Gantry Out"=w505:refnum<k24>)  [unwired: 7 in]
                          n179 = local read "maximum is best focus"() -> (w499:dbl)
                          n180 = Delete From Array(array=w504, index=2) -> (deleted portion=w502:dbl)  [unwired: 1 in, 1 out]
                          n181 = Build Array(w499, w502) -> (w498:dbl[])
                          n182 = Build Array(w498) -> (w497:dbl[][])
                        }
                      }
                    }
                    frame #2 {
                      n183 = call "Z Go.vi"("Increment"=TRUE, "Return Immediately"=FALSE ("Increment"), "error in (no error)"=w508, "Speed In"=1.0 ("Speed"), "Position In"=0.01, "Gantry In"=w511) -> ("error out"=w509:errorcluster, "Gantry Out"=w510:refnum<k24>)  [unwired: 2 in, 2 out]
                    }
                  }
                }
                n184 = Transpose 2D Array(2D array=w466) -> (transposed array=w465:dbl[][])
                n185 = Index Array(array=w465) -> (element #1=w440:dbl[], element #2=w464:dbl[])  [unwired: 4 in]
                n186 = Empty Array?(array=w440) -> (empty?=w439:bool)
                n187 = Array Max & Min(array=w440) -> (max index (indices)=w441:i32)  [unwired: 3 out]
                n188 = case shown="False" w439 {
                  tunnel: w464 -> [w469 _]
                  tunnel: w441 -> [w468 _]
                  tunnel: [w467 w470] -> w453
                  tunnel: w444 -> [_ w472]
                  frame False {
                    n189 = Index Array(array=w469, index=w468) -> (element=w467:dbl)
                  }
                  frame True {
                    n190 = Index Array(array=w472, index=2) -> (element=w470:dbl)
                  }
                }
                n191 = call "Z Go.vi"("Increment"=FALSE, "Return Immediately"=FALSE ("Increment"), "error in (no error)"=w454, "Speed In"=15.0 ("Speed"), "Position In"=w453, "Gantry In"=w452) -> ("error out"=w451:errorcluster, "Gantry Out"=w450:refnum<k24>)  [unwired: 2 in, 2 out]
              }
              frame True {
              }
            }
          }
          frame #2 {
            n192 = local read "Left Fiducial"() -> (w520:dbl[])
            n193 = Empty Array?(array=w520) -> (empty?=w519:bool)
            n194 = case shown="True" w524 {
              tunnel: [w528 w542] -> w522
              tunnel: w525 -> [w529 w539]
              tunnel: w523 -> [w528 w540]
              tunnel: [w527 w538] -> w521
              tunnel: w519 -> [w526 w537]
              frame False {
                n195 = case shown="False" w526 {
                  selector: w526 -> [_ w534]
                  tunnel: w529 -> [w531 w535]
                  tunnel: [w530 w533] -> w527
                  frame False {
                    n196 = property on="Record Top Right" class="Bool (strict)"(error in=w531, "Val(Sgnl)"=TRUE ("Value (Signaling)")) -> (error out=w530:errorcluster)  [unwired: 1 in, 1 out]
                  }
                  frame True {
                    n197 = property on="Record Top Left" class="Bool (strict)"(error in=w535, "Val(Sgnl)"=w534) -> (error out=w533:errorcluster)  [unwired: 1 in, 1 out]
                  }
                }
              }
              frame True {
                n198 = case shown="True" w537 {
                  frame False {
                    n199 = property on="Record Top Right" class="Bool (strict)"("DisabledEnum"=T7."Enabled" ("Disabled")) -> ()  [unwired: 2 in, 2 out]
                    n200 = property on="Record Top Left" class="Bool (strict)"("DisabledEnum"=T7."Disabled and Grayed Out" ("Disabled")) -> ()  [unwired: 2 in, 2 out]
                    n201 = property on="Instructions" class="Str"("Val(Sgnl)"="Use the joystick to match the pattern recognition until a stable red circle appears. \nUse Z controls to focus or override camera presets if needed. \nClick Record Top Right.") -> ()  [unwired: 2 in, 2 out]
                  }
                  frame True {
                    n202 = property on="Record Top Left" class="Bool (strict)"("DisabledEnum"=T7."Enabled" ("Disabled")) -> ()  [unwired: 2 in, 2 out]
                    n203 = property on="Record Top Right" class="Bool (strict)"("DisabledEnum"=T7."Disabled and Grayed Out" ("Disabled")) -> ()  [unwired: 2 in, 2 out]
                    n204 = property on="Instructions" class="Str"("Val(Sgnl)"="Use the joystick to match the pattern recognition until a stable red circle appears.\nUse Z controls to focus or override camera presets if needed. \nClick Record Top Left.") -> ()  [unwired: 2 in, 2 out]
                  }
                }
                n205 = call "Joystick.vi"("error in (no error)"=w539, "Joystick"=TRUE, "Gantry In"=w540) -> ("error out"=w538:errorcluster, "Gantry Out"=w542:refnum<k24>)  [unwired: 7 in]
                n206 = One Button Dialog(message="Warning: Focus failed. Find fiducial manually with joystick. See instructions for more information.") -> ()  [unwired: 1 in, 1 out]
              }
            }
          }
        }
      }
      event "Calculate": Value Change {
        n207 = event-data() -> ()  [unwired: 1 in, 6 out]
        n208 = disable-structure shown="Enabled" {
          frame Disabled {
            n209 = control-ref of="Position Number"() -> (w704:refnum<vi>)
            n210 = property class="DigNum (strict)"(reference=w704, "Val(Sgnl)"=i16 1 ("Value (Signaling)")) -> ()  [unwired: 1 in, 2 out]
          }
          frame Enabled {
          }
        }
        n211 = Unbundle By Name "Unbundle By Name"(w564) -> ("Camera Fiducials"=w567:dbl[][], "Relative Coordinates"=w568:dbl[][], "Assembly Type"=w562:string, "Protomodule?"=w556:bool)  [unwired: 1 out]
        n212 = case shown="\"Module HD Full\"" w562 {
          tunnel: ["Calculate_Centers" ("function name") "Calculate_Centers" ("function name") "Calculate_Centers" ("function name") "Calculate_Centers" ("function name") "Calculate_Centers_Right_Partial" ("function name") "Calculate_Centers_Right_Partial" ("function name")] -> w566
          frame "Protomodule LD Full", Default {
          }
          frame "Protomodule HD Full" {
          }
          frame "Module LD Full" {
          }
          frame "Module HD Full" {
          }
          frame "Module LD Right" {
          }
          frame "Protomodule LD Right" {
          }
        }
        n213 = property on="Calculate" class="Bool (strict)"(error in=w560, "Value"=FALSE ("Calculate")) -> (error out=w559:errorcluster)  [unwired: 1 in, 1 out]
        n214 = Build Array(w567, w568) -> (w565:dbl[][][])
        n215 = for {
          tunnel: w565 -> [w692] mode=indexing
          shift-right: [w690] -> w558
          shift-left: w559 -> [w691]
          tunnel: [w688] -> w555 mode=indexing
          n216 = Array Subset(array=w692, index (row)=0 ("index"), length (row)=2 ("length"), index (col)=0 ("index"), length (col)=2 ("length")) -> (w695:dbl[][])
          n217 = Index Array(array=w695) -> (element #1=w694:dbl[], element #2=w693:dbl[])  [unwired: 4 in]
          n218 = Array To Cluster(array=w694) -> (cluster=w698:cluster{"[0]":dbl, "[1]":dbl})
          n219 = Array To Cluster(array=w693) -> (cluster=w697:cluster{"[0]":dbl, "[1]":dbl})
          n220 = Build Array(w698, w697) -> (w696:cluster{"[0]":dbl, "[1]":dbl}[])
          n221 = call "IMAQ Point Distances"("Points"=w696, "error in (no error)"=w691) -> ("Distances"=w689:sgl[], "error out"=w690:errorcluster)  [unwired: 3 in]
          n222 = Index Array(array=w689) -> (element=w688:sgl)  [unwired: 1 in]
        }
        n223 = Index Array(array=w555) -> (element #1=w554:sgl, element #2=w553:sgl)  [unwired: 2 in]
        n224 = Subtract(x=w554, y=w553) -> (x-y=w552:sgl)
        n225 = Absolute Value(x=w552) -> (abs(x)=w551:sgl)
        n226 = Less?(x=w551, y=sgl 0.02) -> (x < y?=w549:bool)
        "Distance as expected?" <- w549
        n227 = case shown="True" w549 {
          tunnel: w568 -> [_ w594]
          tunnel: w566 -> [_ w590]
          tunnel: w567 -> [_ w588]
          tunnel: w564 -> [w573 w587]
          tunnel: [w573 w582] -> w563
          tunnel: w558 -> [w571 w581]
          tunnel: [w570 w578] -> w557
          tunnel: w556 -> [_ w577]
          frame False {
            n228 = property on="Enter Manual Mode" class="Bool (strict)"(error in=w571, "Val(Sgnl)"=TRUE ("Value (Signaling)")) -> (error out=w570:errorcluster)  [unwired: 1 in, 1 out]
            n229 = One Button Dialog(message="Error: Distance between fiducials does not match expected.\nReview fiducials manually.") -> ()  [unwired: 1 in, 1 out]
          }
          frame True {
            n230 = call "Get Python Version.vi"("error in (no error)"=w581) -> ("Python Version"=w602:string, "error out"=w603:errorcluster)  [unwired: 9 in]
            n231 = Open Python Session(python version=w602, 3:w603) -> (session out=w595:refnum<k35>, error out=w597:errorcluster)  [unwired: 1 in]
            n232 = call "Base File Path.vi"() -> ("Paths Out"=w599:T8)  [unwired: 11 in]
            n233 = Unbundle By Name(w599) -> ("Carrier Tray Folder"=w600:path)
            n234 = Build Path(base path=w600, name or relative path=path "Calculate Baseplate Center.py") -> (appended path=w601:path)
            n235 = Delete From Array(array=w594, length=2, index (row)=7) -> (deleted portion=w576:dbl[][], array with subset deleted=w604:dbl[][])  [unwired: 1 in]
            n236 = node "Python Node"(w595, w601, w590, w597, dbl[][] [], w588, w604) -> (w596:refnum<k35>, w598:errorcluster, w575:dbl[][])  [unwired: 2 in, 2 out]
            n237 = Close Python Session(session in=w596, error in=w598) -> (11:w580:errorcluster)
            n238 = Bundle By Name(cluster=w587, "XYZTheta Centers"=w575, "Pedestal Heights"=w576) -> (w583:T4)
            n239 = flat-sequence {
              tunnel: w583 -> [w613]
              tunnel: [w613] -> w586
              tunnel: w575 -> [w610]
              tunnel: w580 -> [w608]
              tunnel: [w607] -> w579
              tunnel: w586 -> [w615]
              tunnel: [w615] -> w585
              tunnel: [w614] -> w584
              tunnel: [w621] -> w582
              tunnel: w585 -> [w622]
              tunnel: w584 -> [w628]
              tunnel: w579 -> [w627]
              tunnel: [w626] -> w578
              tunnel: w577 -> [w625]
              tunnel: w576 -> [w624]
              tunnel: w575 -> [w623]
              frame #0 {
                n240 = local read "Position Number"() -> (w606:i16)
                n241 = call "even odd check.vi"("position"=w606) -> ("index"=w605:i32)  [unwired: 10 in]
                n242 = Index Array "Index Array"(array=w610, index (row)=w605) -> (element=w609:dbl[])  [unwired: 1 in]
                n243 = Reshape Array "Reshape Array"(w609, u32 4) -> (w612:dbl[])
                n244 = property on="Center" class="Arr (strict)"(error in=w608, "Val(Sgnl)"=w612) -> (error out=w607:errorcluster)  [unwired: 1 in, 1 out]
              }
              frame #1 {
                n245 = disable-structure shown="Enabled" {
                  disable-tunnel: [w616 TRUE ("T button?")] -> w614
                  frame Disabled {
                    n246 = Two Button Dialog(message="Ready to Submit?", 1:"No" ("F button name (\"Cancel\")"), 2:"Yes" ("T button name (\"OK\")")) -> (T button?=w616:bool)
                  }
                  frame Enabled {
                  }
                }
              }
              frame #2 {
                n247 = case shown="True" w628 {
                  tunnel: w627 -> [w630 w639]
                  tunnel: [w631 w638] -> w626
                  tunnel: w625 -> [_ w637]
                  tunnel: w624 -> [_ w636]
                  tunnel: w623 -> [_ w635]
                  tunnel: w622 -> [w629 w634]
                  tunnel: [w629 w633] -> w621
                  frame False {
                    n248 = property on="Enter Manual Mode" class="Bool (strict)"(error in=w630, "Val(Sgnl)"=TRUE ("Value (Signaling)")) -> (error out=w631:errorcluster)  [unwired: 1 in, 1 out]
                  }
                  frame True {
                    n249 = case shown="True" w637 {
                      selector: w637 -> [_ w648]
                      tunnel: w639 -> [w642 w650]
                      tunnel: [w641 w649] -> w638
                      tunnel: w636 -> [_ w647]
                      tunnel: w635 -> [_ w646]
                      tunnel: w634 -> [w640 w645]
                      tunnel: [w640 w644] -> w633
                      frame False {
                        n250 = property on="Auto Submit" class="Bool (strict)"(error in=w642, "Val(Sgnl)"=TRUE ("Value (Signaling)")) -> (error out=w641:errorcluster)  [unwired: 1 in, 1 out]
                      }
                      frame True {
                        n251 = disable-structure shown="Enabled" {
                          disable-tunnel: w650 -> [w662 w687]
                          disable-tunnel: [w661 w686] -> w649
                          disable-tunnel: w648 -> [w660 w685]
                          disable-tunnel: w647 -> [w659 _]
                          disable-tunnel: w646 -> [w658 _]
                          disable-tunnel: w645 -> [w653 w684]
                          disable-tunnel: [w652 w684] -> w644
                          frame Disabled {
                            n252 = disable-structure shown="Enabled" {
                              disable-tunnel: ["component thickness" 1.35 ("component thickness")] -> w654
                              frame Disabled {
                              }
                              frame Enabled {
                              }
                            }
                            n253 = property on="BP check" class="Bool (strict)"(error in=w662, "Val(Sgnl)"=w660) -> (error out=w661:errorcluster)  [unwired: 1 in, 1 out]
                            n254 = Array Subset(array=w658, index (row)=2 ("index"), length (row)=2 ("length")) -> (w655:dbl[][])  [unwired: 2 in]
                            n255 = for {
                              tunnel: w659 -> [w677] mode=indexing
                              tunnel: w655 -> [w675] mode=indexing
                              tunnel: w654 -> [w673]
                              tunnel: [w672] -> w651 mode=indexing
                              i -> [w669]
                              w671 = 2
                              n256 = Equal To 0?(x=w669) -> (x = 0?=w668:bool)
                              n257 = Index Array(array=w677, index=w671) -> (element=w676:dbl)
                              n258 = Select(t=0.5, s=w668, f=-0.5) -> (s? t:f=w665:dbl)
                              n259 = Add(x=w673, y=w676) -> (x+y=w674:dbl)
                              n260 = in-place {
                                in-place-border: w674 -> [w682]
                                in-place-border: w665 -> [w679]
                                n261 = in-place-array #3(w675, w671, 0) -> (w683:dbl, w680:dbl)
                                n262 = Subtract(x=w683, y=w682) -> (x-y=w681:dbl)
                                n263 = Add(x=w680, y=w679) -> (x+y=w678:dbl)
                                n264 = in-place-array #3(w681, w678) -> (w672:dbl[])  [unwired: 2 out]
                              }
                            }
                            n265 = Bundle By Name(cluster=w653, "Offset pins"=w651) -> (w652:T4)
                          }
                          frame Enabled {
                            n266 = property on="Auto Submit" class="Bool (strict)"(error in=w687, "Val(Sgnl)"=w685) -> (error out=w686:errorcluster)  [unwired: 1 in, 1 out]
                          }
                        }
                      }
                    }
                  }
                }
              }
            }
          }
        }
      }
      event "BP check": Value Change {
        n267 = event-data() -> ()  [unwired: 1 in, 6 out]
        n268 = flat-sequence {
          frame #0 {
            n269 = local write "Machine Vision"(Machine_Vision."None" ("Machine Vision")) -> ()
          }
          frame #1 {
            n270 = property on="BP check" class="Bool (strict)"("Value"=FALSE ("BP check")) -> ()  [unwired: 2 in, 2 out]
          }
        }
        n271 = Unbundle By Name(w711) -> ("XYZTheta Centers"=w725:dbl[][], "Offset pins"=w719:dbl[][])
        n272 = Array Subset(array=w725, index (row)=0 ("index"), length (row)=2 ("length")) -> (w722:dbl[][])  [unwired: 2 in]
        n273 = for {
          tunnel: w722 -> [w774] mode=indexing
          shift-right: [w758] -> w714
          shift-left: w721 -> [w739]
          shift-right: [w752] -> w718
          shift-left: w720 -> [w738]
          tunnel: w719 -> [w763] mode=indexing
          tunnel: [w751] -> w712 mode=indexing
          w749 = 300.0 ("Speed")
          n274 = Index Array(array=w763) -> (element #1=w768:dbl, element #2=w767:dbl, element #3=w750:dbl)  [unwired: 3 in]
          n275 = Build Array(w768, w767) -> (w766:dbl[])
          n276 = Replace Array Subset(array=w774, new element=w750, index=2) -> (w747:dbl[])
          n277 = Index Array(array=w747) -> (element #1=w745:dbl, element #2=w744:dbl, element #3=w742:dbl)  [unwired: 3 in]
          n278 = Build Array(w745, w744) -> (w743:dbl[])
          n279 = call "Z Go.vi"("Increment"=FALSE, "error in (no error)"=w738, "Speed In"=15.0, "Position In"=w742, "Gantry In"=w739) -> ("error out"=w737:errorcluster, "Gantry Out"=w736:refnum<k24>)  [unwired: 3 in, 2 out]
          n280 = call "XY Go.vi"("Increment?"=FALSE, "error in (no error)"=w737, "Speed"=w749, "XY In"=w743, "Gantry In"=w736) -> ("error out"=w734:errorcluster, "Gantry Out"=w735:refnum<k24>)  [unwired: 4 in, 1 out]
          n281 = call "Focus BP.vi"("error in"=w734, "Scan Inc"=0.01, "Start Inc"=-0.1, "Gantry In"=w735) -> ("error out"=w761:errorcluster, "max value"=w754:dbl, "Gantry Out"=w762:refnum<k24>)  [unwired: 5 in]
          n282 = call "XY Go.vi"("Increment?"=FALSE, "error in (no error)"=w761, "Speed"=w749, "XY In"=w766, "Gantry In"=w762) -> ("error out"=w770:errorcluster, "Gantry Out"=w771:refnum<k24>)  [unwired: 4 in, 1 out]
          n283 = call "Z Go.vi"("Increment"=FALSE, "error in (no error)"=w770, "Speed In"=15.0, "Position In"=w750, "Gantry In"=w771) -> ("error out"=w759:errorcluster, "Gantry Out"=w760:refnum<k24>)  [unwired: 3 in, 2 out]
          n284 = call "Focus BP.vi"("error in"=w759, "Scan Inc"=0.01, "Start Inc"=-0.1, "Gantry In"=w760) -> ("error out"=w752:errorcluster, "max value"=w753:dbl, "Gantry Out"=w758:refnum<k24>)  [unwired: 5 in]
          n285 = Subtract(x=w754, y=w753) -> (x-y=w757:dbl)
          n286 = Absolute Value(x=w757) -> (abs(x)=w756:dbl)
          n287 = Less?(x=w756, y=0.1) -> (x < y?=w751:bool)
        }
        n288 = And Array Elements(Boolean array=w712) -> (logical AND=w713:bool)
        n289 = case shown="True" w713 {
          selector: w713 -> [_ w733]
          tunnel: w718 -> [w728 w732]
          tunnel: [w727 w733] -> w717
          tunnel: [w726 w732] -> w716
          frame False {
            n290 = while {
              shift-right: [w730] -> w726
              shift-left: w728 -> [w731]
              tunnel: [w729] -> w727
              stop <- w729 stop-if-true
              n291 = call "Prompt User for Input2"("error in (no error)"=w731) -> ("Baseplate ready?"=w729:bool, "error out"=w730:errorcluster)  [unwired: 16 in, 1 out]
            }
          }
          frame True {
          }
        }
        n292 = property on="Auto Submit" class="Bool (strict)"(error in=w716, "Val(Sgnl)"=w717) -> (error out=w715:errorcluster)  [unwired: 1 in, 1 out]
      }
      event "Go to Center", "Position Number": Value Change {
        n293 = event-data() -> ()  [unwired: 1 in, 6 out]
        n294 = Unbundle By Name(w790) -> ("XYZTheta Centers"=w783:dbl[][])
        n295 = call "even odd check.vi"("position"="Position Number") -> ("index"=w779:i32)  [unwired: 10 in]
        n296 = Index Array "Index Array"(array=w783, index (row)=w779) -> (element=w785:dbl[])  [unwired: 1 in]
        n297 = Reshape Array "Reshape Array"(w785, u32 4) -> (w782:dbl[])
        n298 = case shown="True" "Go to Center" {
          tunnel: w782 -> [w791 w800]
          tunnel: w790 -> [w793 w802]
          tunnel: [w793 w802] -> w789
          tunnel: w787 -> [w792 w796]
          tunnel: [w792 w801] -> w784
          frame False {
            # "Change Position Number"
            "Center" <- w791
          }
          frame True {
            n299 = control-ref of="Joystick"() -> (w799:refnum<vi>)
            n300 = property class="Bool (strict)"(reference=w799) -> (reference out=w797:refnum<vi>, "Value"=w798:bool)  [unwired: 1 in, 1 out]
            n301 = case shown="True" w798 {
              selector: w798 -> [_ w808]
              tunnel: w796 -> [w803 w807]
              tunnel: [w803 w806] -> w795
              tunnel: w797 -> [_ w804]
              frame False {
              }
              frame True {
                n302 = Not(x=w808) -> (.not. x?=w805:bool)
                n303 = property class="Bool (strict)"(reference=w804, "Value"=w805) -> ()  [unwired: 1 in, 2 out]
                n304 = call "Joystick.vi"("Joystick"=w805, "Gantry In"=w807) -> ("Gantry Out"=w806:refnum<k24>)  [unwired: 8 in, 1 out]
              }
            }
            n305 = call "ClearXYZTheta Go.vi"("Speed"=300.0, "XYZTheta In"=w800, "Gantry In"=w795) -> ("Gantry Out"=w801:refnum<k24>)  [unwired: 6 in, 2 out]
          }
        }
      }
      event "Stop", "Auto Submit": Value Change {
        n306 = event-data() -> ()  [unwired: 1 in, 6 out]
        n307 = flat-sequence {
          frame #0 {
          }
          frame #1 {
            n308 = property on="Auto Submit" class="Bool (strict)"("Value"=FALSE ("Auto Submit")) -> ()  [unwired: 2 in, 2 out]
          }
        }
        n309 = property on="Both fiducials recorded" class="Bool (strict)"() -> ("Value"=w815:bool)  [unwired: 2 in, 2 out]
        n310 = property on="Stop" class="Bool"("DisabledEnum"=T7."Enabled" ("Disabled")) -> ()  [unwired: 2 in, 2 out]
        n311 = case shown="True" w815 {
          selector: w815 -> [w872 _]
          tunnel: [w872 w874] -> w810
          frame False {
            n312 = One Button Dialog(message="At least one fiducial not recorded!") -> ()  [unwired: 1 in, 1 out]
          }
          frame True {
            n313 = property on="Distance as expected?" class="Bool (strict)"() -> ("Value"=w875:bool)  [unwired: 2 in, 2 out]
            n314 = case shown="True" w875 {
              selector: w875 -> [w876 w878]
              tunnel: [w876 w878] -> w874
              frame False {
                n315 = One Button Dialog(message="Distance between fiducials does not match expected. Find fiducials again.") -> ()  [unwired: 1 in, 1 out]
              }
              frame True {
              }
            }
          }
        }
        "Program Done?" <- w810
        n316 = case shown="True" w810 {
          tunnel: w814 -> [w818 w850]
          tunnel: w813 -> [w819 w848]
          tunnel: [w819 w846] -> w812
          tunnel: [w818 w843] -> w811
          tunnel: w809 -> [_ w839]
          frame False {
          }
          frame True {
            n317 = Unbundle By Name(w839) -> ("Fiducials"=w838:path, "Gantry Fiducials"=w824:dbl[], "avg value count"=w833:dbl[], "Previous Avgs"=w837:dbl[][])
            n318 = call "Joystick.vi"("error in (no error)"=w850, "Joystick"=FALSE, "Gantry In"=w848) -> ("error out"=w851:errorcluster, "Gantry Out"=w846:refnum<k24>)  [unwired: 7 in]
            n319 = in-place {
              in-place-border: [w855] -> w832
              in-place-border: [w854] -> w831
              n320 = in-place-array #4(w833, 0) -> (w855:dbl)
              n321 = Increment(x=w855) -> (x+1=w854:dbl)
              n322 = in-place-array #4(w854) -> (w829:dbl[])  [unwired: 1 out]
            }
            n323 = Index Array(array=w824, index #1=2 ("index"), index #2=5 ("index")) -> (element #1=w821:dbl, element #2=w820:dbl)
            n324 = Multiply(x=w837, y=w832) -> (x*y=w842:dbl[][])
            n325 = Reshape Array(w824, 2 ("dimension size"), 3 ("dimension size")) -> (w834:dbl[][])
            n326 = for {
              tunnel: w834 -> [w859] mode=indexing
              tunnel: w842 -> [w860] mode=indexing
              tunnel: w831 -> [w857]
              tunnel: [w856] -> w841 mode=indexing
              n327 = Add(x=w859, y=w860) -> (x+y=w858:dbl[])
              n328 = Divide(x=w858, y=w857) -> (x/y=w856:dbl[])
            }
            n329 = Reshape Array(w841, 6 ("dimension size")) -> (w827:dbl[])
            n330 = in-place {
              in-place-border: w821 -> [w853]
              in-place-border: w820 -> [w852]
              n331 = in-place-array #5(w827, 2, 5) -> ()  [unwired: 2 out]
              n332 = in-place-array #5(w853, w852) -> (w825:dbl[])  [unwired: 2 out]
            }
            n333 = call "Replace Row In File.vi"("error in"=w851, "Index"=0, "Insert Array"=w825, "Path"=w838) -> ("error out"=w844:errorcluster)  [unwired: 7 in]
            n334 = call "Replace Row In File.vi"("error in"=w844, "Index"=1, "Insert Array"=w829, "Path"=w838) -> ("error out"=w843:errorcluster)  [unwired: 7 in]
          }
        }
        n335 = disable-structure shown="Enabled" {
          disable-tunnel: w811 -> [w862 w871]
          disable-tunnel: [_ w871] -> w817
          frame Disabled {
            n336 = case shown="No Error" w862 {
              tunnel: "Fiducial" -> [w863 w870]
              frame No Error {
                w864 = "\r"
                n337 = Concatenate Strings("Success!", w864, w864, w863, " Values Stored") -> ()  [unwired: 1 out]
              }
              frame Error {
                w867 = "\r"
                n338 = Concatenate Strings("Error!", w867, w867, w870, " Values Not Stored") -> ()  [unwired: 1 out]
              }
            }
          }
          frame Enabled {
          }
        }
      }
      event "Autofiducial (Beta)": Value Change {
        n339 = event-data() -> ()  [unwired: 1 in, 6 out]
        n340 = disable-structure shown="Enabled" {
          disable-tunnel: [w892 w925] -> w885
          disable-tunnel: w884 -> [w891 w925]
          disable-tunnel: "Autofiducial (Beta)" -> [w890 _]
          disable-tunnel: w881 -> [w888 _]
          disable-tunnel: [w886 _] -> w880
          frame Enabled {
            n341 = flat-sequence {
              tunnel: w890 -> [_]
              tunnel: [w898] -> w889
              tunnel: w891 -> [w903]
              tunnel: [w903] -> w897
              tunnel: [w902] -> w896
              tunnel: [w901] -> w895
              tunnel: w889 -> [w900]
              tunnel: w897 -> [w910]
              tunnel: [w909] -> w894
              tunnel: w896 -> [w908]
              tunnel: [w907] -> w893
              tunnel: w895 -> [w907]
              tunnel: w888 -> [w906]
              tunnel: [w904] -> w887
              tunnel: [w919] -> w892
              tunnel: w894 -> [w920]
              tunnel: w893 -> [w918]
              tunnel: w887 -> [w917]
              tunnel: [w915] -> w886
              frame #0 {
                n342 = local read "Image"() -> (w899:T5)
                n343 = call "Find Fiducial.vi"("Image"=w899) -> ("Move by (mm)"=w898:dbl[])  [unwired: 3 in]
              }
              frame #1 {
                n344 = Index Array(array=w900) -> (element #1=w902:dbl, element #2=w901:dbl)  [unwired: 2 in]
                "Move by" <- w900
              }
              frame #2 {
                n345 = call "Joystick.vi"("error in (no error)"=w906, "Joystick"=FALSE, "Gantry In"=w910) -> ("error out"=w905:errorcluster, "Gantry Out"=w911:refnum<k24>)  [unwired: 7 in]
                n346 = call "Move Inc.vi"("Axis"="X", "error in (no error)"=w905, "Speed"=25.0, "Distance"=w908, "Gantry In"=w911) -> ("error out"=w904:errorcluster, "Gantry Out"=w909:refnum<k24>)  [unwired: 5 in]
              }
              frame #3 {
                n347 = call "Joystick.vi"("error in (no error)"=w917, "Joystick"=FALSE, "Gantry In"=w920) -> ("error out"=w916:errorcluster, "Gantry Out"=w921:refnum<k24>)  [unwired: 7 in]
                n348 = call "Move Inc.vi"("Axis"="Y", "error in (no error)"=w916, "Speed"=25.0, "Distance"=w918, "Gantry In"=w921) -> ("error out"=w915:errorcluster, "Gantry Out"=w919:refnum<k24>)  [unwired: 5 in]
              }
            }
          }
          frame Disabled {
          }
        }
      }
    }
    n349 = Equal?(x=w94, y=0) -> (x = y?=w92:bool)
    n350 = case shown="True" w92 {
      selector: w92 -> [_ w108]
      tunnel: w91 -> [_ w103]
      frame False {
      }
      frame True {
        w107 = T7."Disabled and Grayed Out" ("Disabled")
        n351 = property on="Go to Top Left Fiducial" class="Bool (strict)"("Val(Sgnl)"=w108) -> ()  [unwired: 2 in, 2 out]
        n352 = Unbundle By Name(w103) -> ("Assembly Type"=w102:string, "Tray Number"=w100:string)  [unwired: 1 out]
        n353 = property on="Stop" class="Bool"("DisabledEnum"=w107) -> ()  [unwired: 2 in, 2 out]
        n354 = Concatenate Strings("Now measuring Tray " ("initial string"), w100, " for " ("string"), w102) -> (→"resulting string":string)
        n355 = property on="Go to Center" class="Bool"("DisabledEnum"=w107) -> ()  [unwired: 2 in, 2 out]
        n356 = property on="Record Top Right" class="Bool (strict)"("DisabledEnum"=w107) -> ()  [unwired: 2 in, 2 out]
        n357 = property on="Go to Top Right Fiducial" class="Bool (strict)"("DisabledEnum"=w107) -> ()  [unwired: 2 in, 2 out]
        n358 = property on="Record Top Left" class="Bool (strict)"("DisabledEnum"=w107) -> ()  [unwired: 2 in, 2 out]
        n359 = property on="Go to Top Left Fiducial" class="Bool (strict)"("DisabledEnum"=w107) -> ()  [unwired: 2 in, 2 out]
        "Instructions" <- "Answer prompts then wait for gantry movement." ("Instructions")
      }
    }
  }
  "Gantry Out" <- w11
  "error out" <- w3
  n360 = Unbundle By Name(w13) -> ("XYZTheta Centers"=→"XYZTheta Centers":dbl[][], "Pedestal Heights"=→"Pedestal Heights":dbl[][])
